vi "HandleDisable.vi"(0 "MenuDisableCol in":refnum<class "MenuDisableCol.lvclass">, 1 "Col Array Ref in":refnum<vi>, 5 "ToDisable in":refnum<class "Column.lvclass">, 7 "Table Data in":string[][](array[string]), 9 "Table CtlRef in":refnum<vi>, 11 "error in (no error)":errorcluster, 12 "Cell Position":T1) -> (4 "MenuDisableCol out":refnum<class "MenuDisableCol.lvclass">, 6 "ToDisable out":refnum<class "Column.lvclass">, 8 "Table Data out":string[][](array[string]), 10 "Table CtlRef Out":refnum<vi>, 15 "error out":errorcluster)   [LabVIEW 2013, in "MenuDisableCol.lvclass"]
uses:
  MenuDisableCol.lvclass
  Column/Column.lvclass
  Globals/DisabledColorGlobal.vi
  <vilib>/Utility/miscctls.llb/LVRowAndColumnTypeDef.ctl
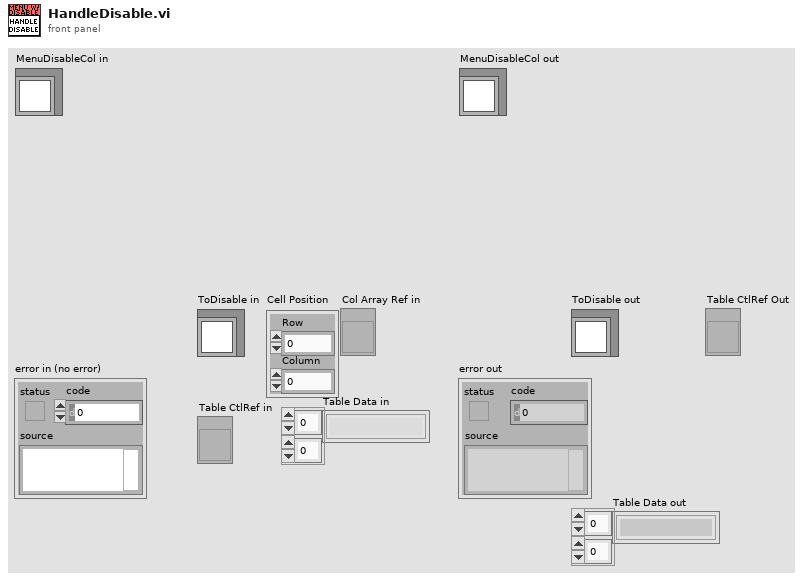
[diagram p1: front panel]
types:
  T1 = typedef "LVRowAndColumnTypeDef.ctl" = cluster{"Row":i32, "Column":i32}
  T2 = typedef "DisableModes.ctl" = u16
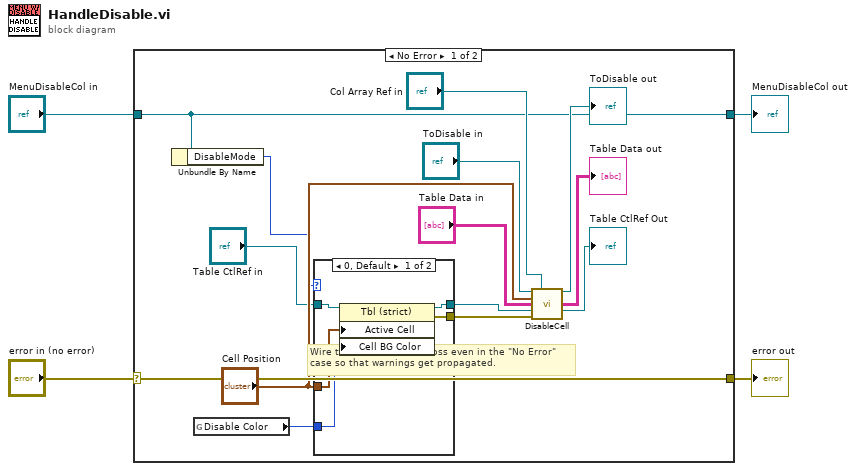
[diagram p0: block diagram]
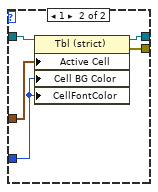
[diagram p2: hidden frame]
diagram:
  n1 = case shown="No Error" "error in (no error)" {
    selector: "error in (no error)" -> [w18 w30]
    tunnel: [w18 w30] -> w3
    tunnel: [w6 w29] -> w1
    tunnel: "MenuDisableCol in" -> [w6 w29]
    frame No Error {
      # "Wire the error cluster across even in the \"No Error\"\ncase so that warnings get propagated."
      n2 = Unbundle By Name(w6) -> ("DisableMode"=w5:T2)
      n3 = global read "DisabledColorGlobal.vi" "Disable Color"() -> (w16:u32)
      n4 = case shown="0, Default" w5 {
        tunnel: [w23 w28] -> w14
        tunnel: [w22 w27] -> w15
        tunnel: w16 -> [w21 w24]
        tunnel: "Cell Position" -> [w20 w26]
        tunnel: "Table CtlRef in" -> [w19 w25]
        frame 0, Default {
          n5 = property class="Tbl (strict)"(reference=w19, "Active Cell"=w20, "Cell BG Color"=w21) -> (reference out=w23:refnum<vi>, error out=w22:errorcluster)  [unwired: 1 in]
        }
        frame 1 {
          n6 = property class="Tbl (strict)"(reference=w25, "Active Cell"=w26, "Cell BG Color"=w24, "CellFontColor"=w24) -> (reference out=w28:refnum<vi>, error out=w27:errorcluster)  [unwired: 1 in]
        }
      }
      n7 = call-dynamic "DisableCell.vi"("Column in"="ToDisable in", "Col Array Ref in"="Col Array Ref in", "Cell Position"="Cell Position", "Table Data in"="Table Data in", "Table CtlRef In"=w14, "error in (no error)"=w15) -> ("Column out"=→"ToDisable out":refnum<class "Column.lvclass">, "Table Data out"=→"Table Data out":string[][], "Table CtlRef Out"=→"Table CtlRef Out":refnum<vi>)  [unwired: 6 in, 1 out]
    }
    frame Error {
    }
  }
  "error out" <- w3
  "MenuDisableCol out" <- w1
